vi "CAlex2_InitAll.vi"(8 "error in (no error)":errorcluster, 10 "LegProperties":T1={"BodyDim"={"ThighLt (m)"=0.4, "ShankLt (m)"=0.41, "HipWd (m)"=0.32}, "BodyWt"={"Thigh (kg)"=0.0, "Shank (kg)"=0.0}, "Cuff Loc"={"HipCuffWd (m)"=0.4, "HipCuffHt (m)"=0.1, "HipFwdShift (m)"=0.0, "ThighToKnee (m)"=0.25, "ThighCuffDist (m)"=0.0, "ShankToKnee (m)"=0.15}}, 11 "CAlex2 in":refnum<class "CAlex2.lvclass">) -> (0 "error out":errorcluster, 3 "CAlex2 out":refnum<class "CAlex2.lvclass">)   [LabVIEW 2015, in "CAlex2.lvclass"]
uses:
  CAlex2.lvclass
  TypeDef/LowerBodyDim.ctl
  SerialChain/xyzO.ctl
  <vilib>/Analysis/Matrix/Datatypes/RealMatrix.ctl
  CAlex2.lvclass/CAlex2.ctl
  SerialChain/SerialChain.lvclass
  <vilib>/Analysis/Matrix/NI_Matrix.lvlib
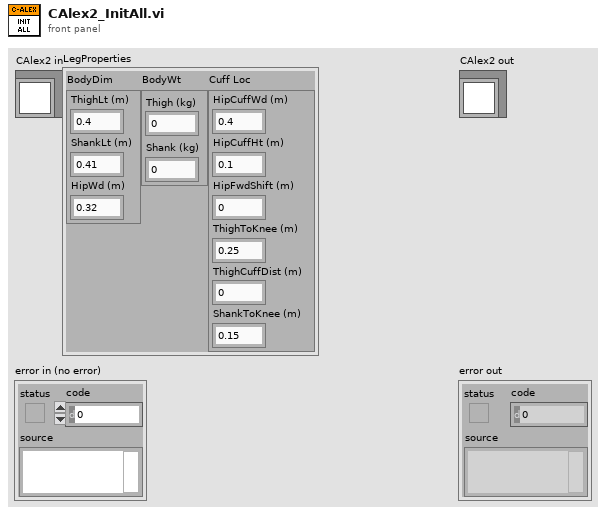
[diagram p1: front panel]
types:
  T1 = typedef "CAlex2.lvclass/LowerBodyDim.ctl" = cluster{"BodyDim":cluster{"ThighLt (m)":dbl, "ShankLt (m)":dbl, "HipWd (m)":dbl}, "BodyWt":cluster{"Thigh (kg)":dbl, "Shank (kg)":dbl}, "Cuff Loc":cluster{"HipCuffWd (m)":dbl, "HipCuffHt (m)":dbl, "HipFwdShift (m)":dbl, "ThighToKnee (m)":dbl, "ThighCuffDist (m)":dbl, "ShankToKnee (m)":dbl}}
  T2 = typedef "NI_Matrix.lvlib/RealMatrix.ctl" = dbl[][]
  T3 = typedef "SerialChain.lvclass/xyzO.ctl" = enum16{"X", "Y", "Z", "O"}
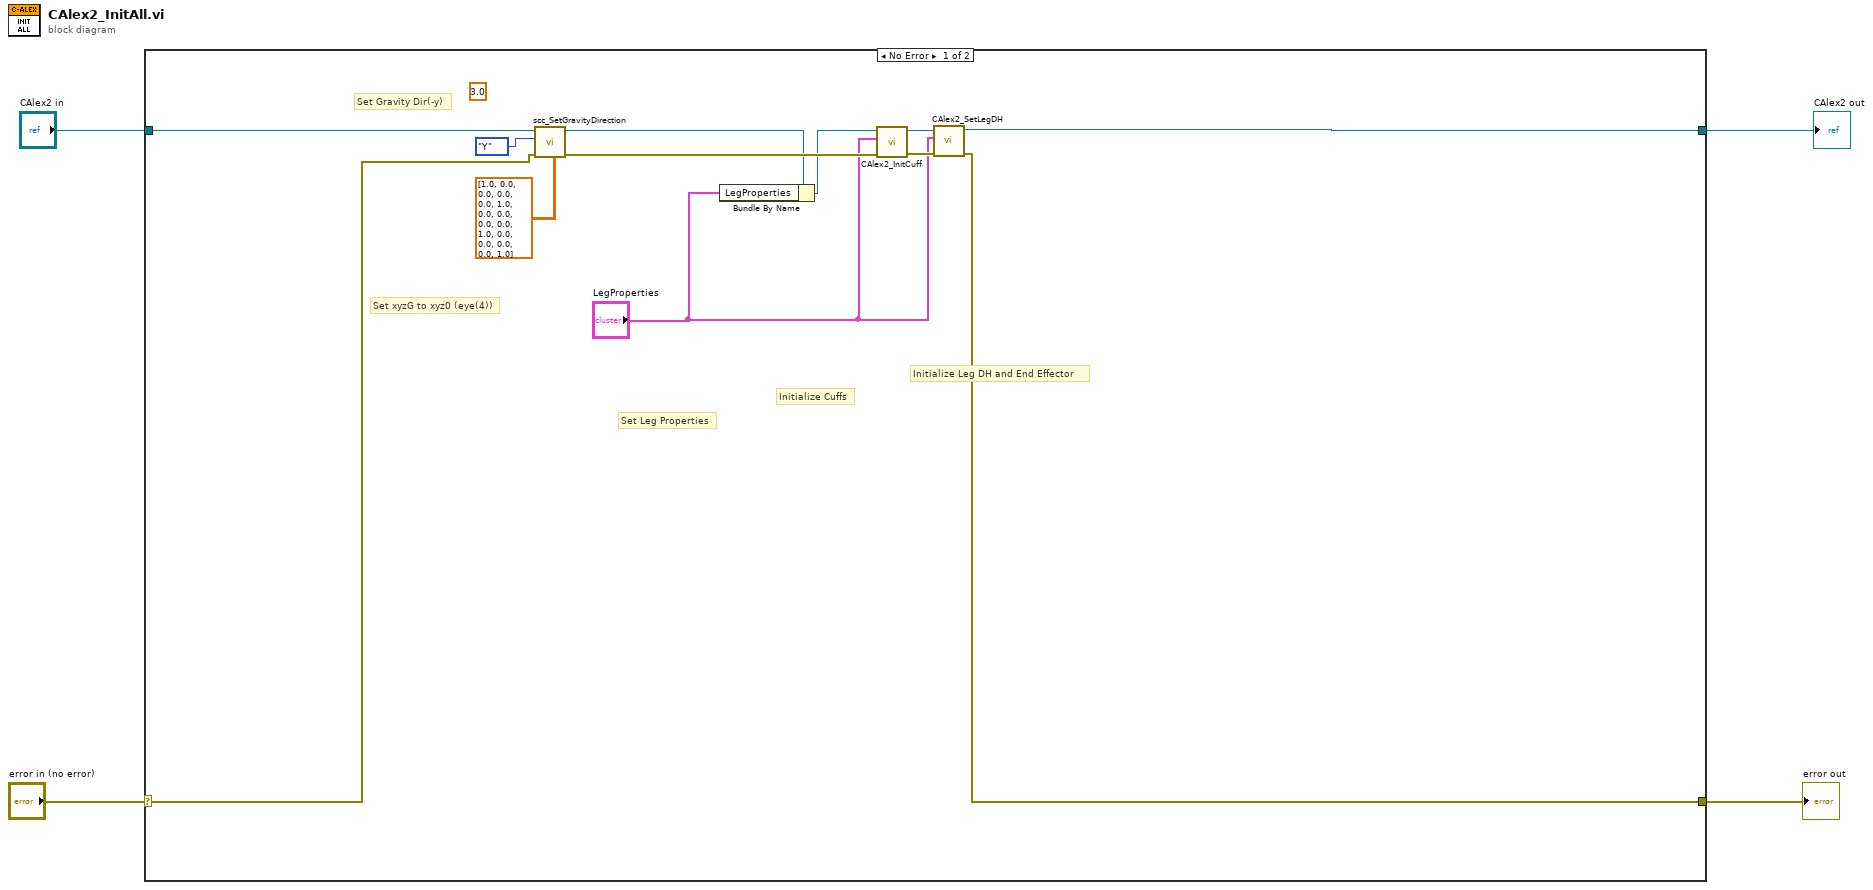
[diagram p0: block diagram]
diagram:
  n1 = case shown="No Error" "error in (no error)" {
    selector: "error in (no error)" -> [w7 w18]
    tunnel: [w6 w18] -> w3
    tunnel: [w13 w17] -> w1
    tunnel: "CAlex2 in" -> [w15 w17]
    frame No Error {
      (unwired) 3.0 ("Numeric")
      # "Initialize Leg DH and End Effector"
      # "Initialize Cuffs"
      # "Set Leg Properties"
      # "Set xyzG to xyz0 (eye(4))"
      # "Set Gravity Dir(-y)"
      n2 = call-dynamic "scc_SetGravityDirection.vi"("Trans_Gto0"=T2 [[1.0, 0.0, 0.0, 0.0], [0.0, 1.0, 0.0, 0.0], [0.0, 0.0, 1.0, 0.0], [0.0, 0.0, 0.0, 1.0]] ("Trans_0toG"), "error in (no error)"=w7, "Gravity Axis in G (Z)"=xyzO."Y" ("Gravity Axis"), "CSC in"=w15) -> ("error out"=w11:errorcluster, "CSC out"=w10:refnum<class "CAlex2.lvclass">)  [unwired: 6 in]
      n3 = Bundle By Name(cluster=w10, "LegProperties"="LegProperties") -> (w8:refnum<class "CAlex2.lvclass">)
      n4 = call-dynamic "CAlex2_InitCuff.vi"("error in (no error)"=w11, "LegProperty"="LegProperties", "CAlex2 in"=w8) -> ("error out"=w12:errorcluster, "CAlex2 out"=w14:refnum<class "CAlex2.lvclass">)  [unwired: 7 in]
      n5 = call-dynamic "CAlex2_SetLegDH.vi"("error in (no error)"=w12, "ArmProperty"="LegProperties", "CAlex2 in"=w14) -> ("error out"=w6:errorcluster, "CAlex2 out"=w13:refnum<class "CAlex2.lvclass">)  [unwired: 7 in]
    }
    frame Error {
    }
  }
  "error out" <- w3
  "CAlex2 out" <- w1
